vi "Process.vi"(8 "error in":errorcluster, 11 "Inst UI.SPC":refnum<class "Inst UI.SPC.lvclass">) -> (0 "error out":errorcluster, 3 "Inst UI.SPC out":refnum<class "Inst UI.SPC.lvclass">)   [LabVIEW 2019, in "Inst UI.SPC.lvclass"]
doc: "---------------------------------------------------------------\nJKI State Machine Objects™\nhttp://jki.net/state-machine-objects/\nCopyright (C) 2005-2015, JKI <info@jki.net>\nALL RIGHTS RESERVEDJKI State Machine Objects (SMO) 1.0.0.5\nJKI - JKI\nCopyright (c) 2016, JKI"
uses:
  Inst UI.SPC.lvclass
  <vilib>/JKI/JKI SMO/SMO/SMO.lvclass
  <vilib>/JKI/JKI SMO/SMO.UI/SMO.UI.lvclass
  <userlib>/LevyLab/Instrument Framework/SMOs/Instrument/Instrument.lvclass
  Inst.SPC/Typedefs/Inst.SPC.getAll--Cluster.ctl
  Inst.SPC/Inst.SPC.lvclass
  <userlib>/LevyLab/Instrument Framework/SMOs/Instrument UI/Instrument UI.lvclass
  Inst UI.SPC.UI--Cluster.ctl
  <userlib>/LevyLab/Instrument Framework/SMOs/Configuration/Configuration.lvclass
  Inst.SPC/Typedefs/Inst.SPC.Configuration--Cluster.ctl
  <userlib>/LevyLab/Instrument Framework/SMOs/Instrument/Typedefs/Client Type--Enum.ctl
  <userlib>/LevyLab/Instrument Framework/SMOs/RemoteControl/Typedefs/Message--Cluster.ctl
  <userlib>/LevyLab/Instrument Framework/SMOs/RemoteControl/RemoteControl.lvclass
  09e9697b-516c-49fb-b2dc-692589121b6f.vi
  C:/Program Files (x86)/National Instruments/LabVIEW 2019/user.lib/LevyLab/Instrument Framework/SMOs/Instrument UI/Instrument UI.lvclass
  C:/Program Files (x86)/National Instruments/LabVIEW 2019/vi.lib/JKI/JKI SMO/SMO.UI/SMO.UI.lvclass
  C:/Program Files (x86)/National Instruments/LabVIEW 2019/vi.lib/JKI/JKI SMO/SMO/SMO.lvclass
  C:/Program Files (x86)/National Instruments/LabVIEW 2019/user.lib/LevyLab/Instrument Framework/Instrument Types/VSource/Instrument.VSource.lvclass
  C:/Program Files (x86)/National Instruments/LabVIEW 2019/user.lib/LevyLab/Instrument Framework/SMOs/Instrument/Instrument.lvclass
panel:
  out "DummyData":string
  out "SPC":string
  out "DCC":string
  in  "GetConfig":bool
  in  "Parameter 2":string
  out "Counter":u32
  in  "Set Parameter":bool
  in  "Parameter":dbl
  in  "STOP":bool
  # "Connected Modules"
  # "DCC"
  # "SPC"
  # "SMO UI Template"
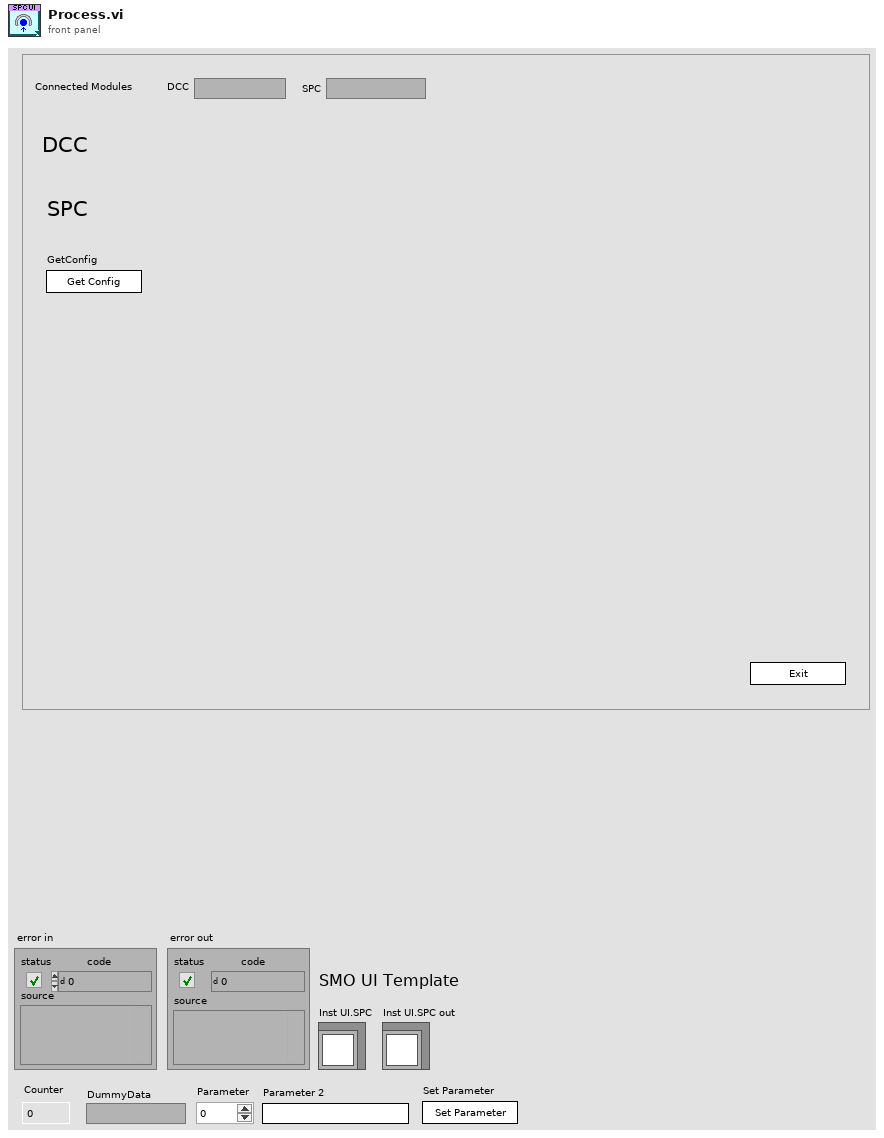
[diagram p1: front panel]
types:
  T1 = typedef "Inst.SPC.lvclass/Inst.SPC.Configuration--Cluster.ctl" = cluster{"DCC_DLL":path, "SPC_DLL":path, "DCC_Serials":string[], "SPC_Serials":string[]}
  T2 = enum32{"invalid app kind", "Development System", "Run Time System", "Student Edition", "Embedded LabVIEW", "Evaluation", "Custom"}
  T3 = enum32{"Invalid", "Standard", "Closed", "Hidden", "Minimized", "Maximized"}
  T4 = typedef "Instrument.lvclass/Client Type--Enum.ctl" = enum16{"Remote", "Local"}
  T5 = typedef "Inst.SPC.lvclass/Inst.SPC.getAll--Cluster.ctl" = cluster{"DummyData":string}
  T6 = typedef "Inst UI.SPC.lvclass/Inst UI.SPC.UI--Cluster.ctl" = cluster{"Parameter":dbl, "Parameter 2":string}
  T7 = typedef "RemoteControl.lvclass/Message--Cluster.ctl" = cluster{"Command":string, "Data":variant, "ID":string}
  T8 = cluster{"Core":cluster{"Current VI Reference":refnum<vi>, "Close Panel on Exit?":bool, "Last Error":cluster{"error":errorcluster, "previous state":string, "remaining states":string}, "Shutdown?":bool}, "Instrument UI":refnum<class "Inst UI.SPC.lvclass">, "Instrument":refnum<class "Inst.SPC.lvclass">, "Configuration":refnum<class "Configuration.lvclass">, "Config Cluster":T1, "getAll":T5, "UI Cluster":T6, "Message":T7}
  T9 = cluster{"Current VI Reference":refnum<vi>, "Close Panel on Exit?":bool, "Last Error":cluster{"error":errorcluster, "previous state":string, "remaining states":string}, "Shutdown?":bool}
  T10 = typedef "SMO.lvclass/Protected Events.ctl" = cluster{"StopProcesses":refnum<user-event>, "AbortProcesses":refnum<user-event>, "Config Changed":refnum<user-event>, "Dependency":refnum<user-event>}
  T11 = typedef "Instrument.lvclass/PublicEvents--Cluster.ctl" = cluster{"MessageFromProcess":refnum<user-event>}
  T12 = typedef "Inst.SPC.lvclass/PublicEvents--Cluster.ctl" = cluster{"MessageFromProcess":refnum<user-event>}
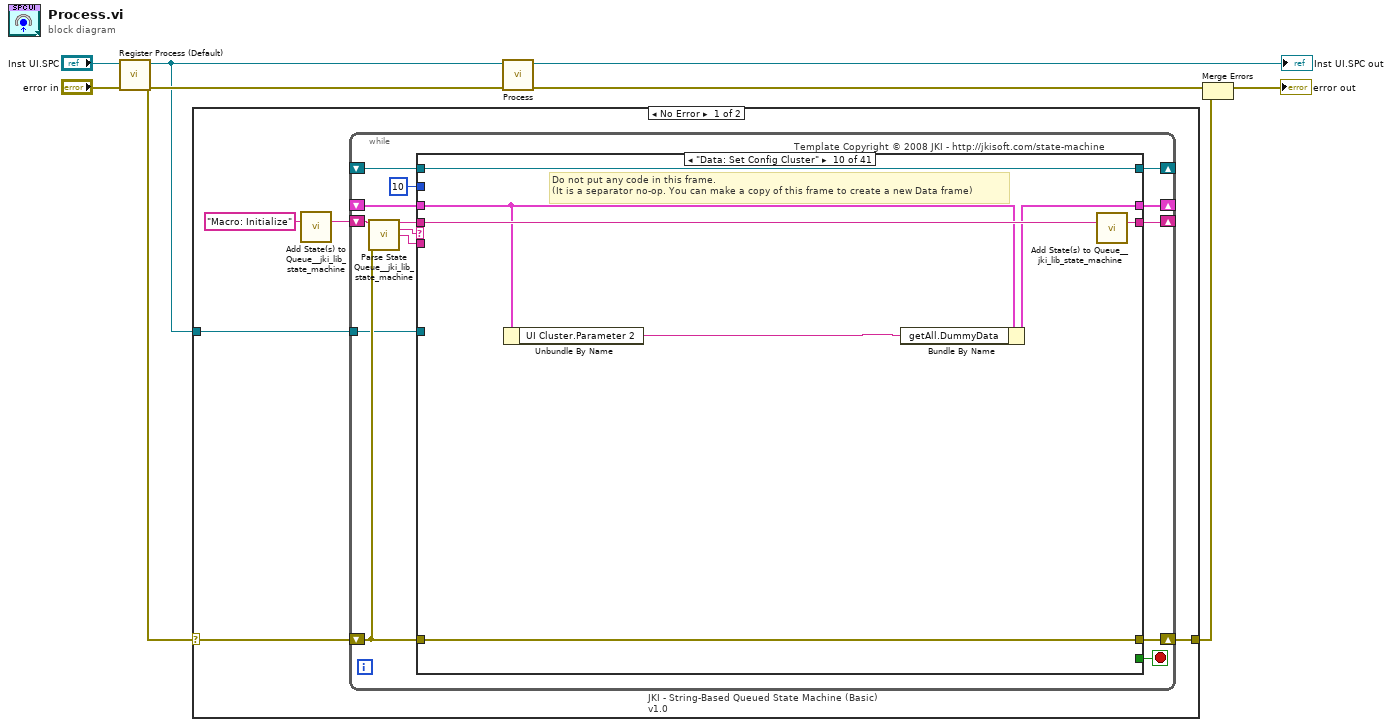
[diagram p0: block diagram]
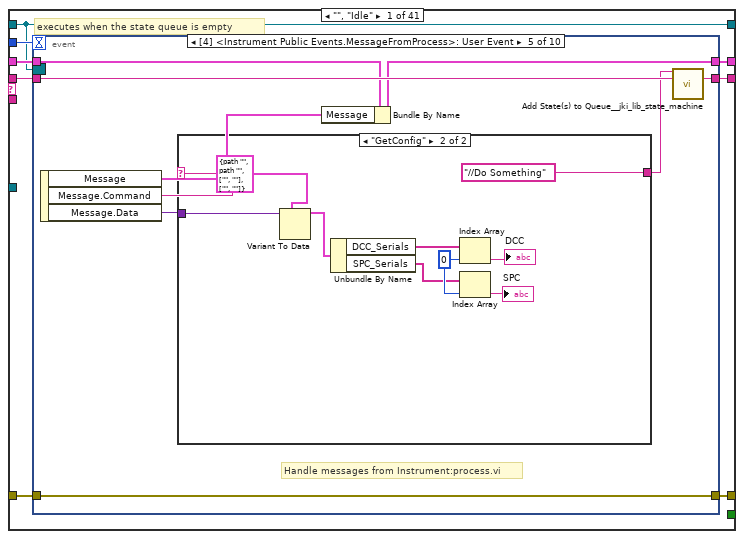
[diagram p2: hidden frame]
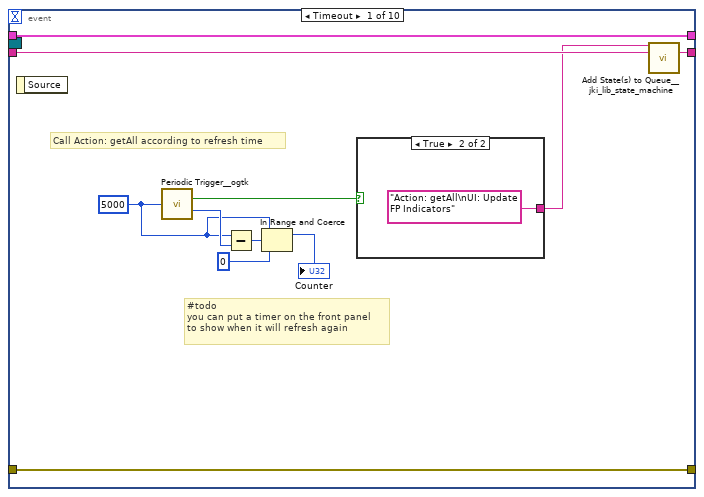
[diagram p3: hidden frame]
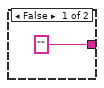
[diagram p4: hidden frame]
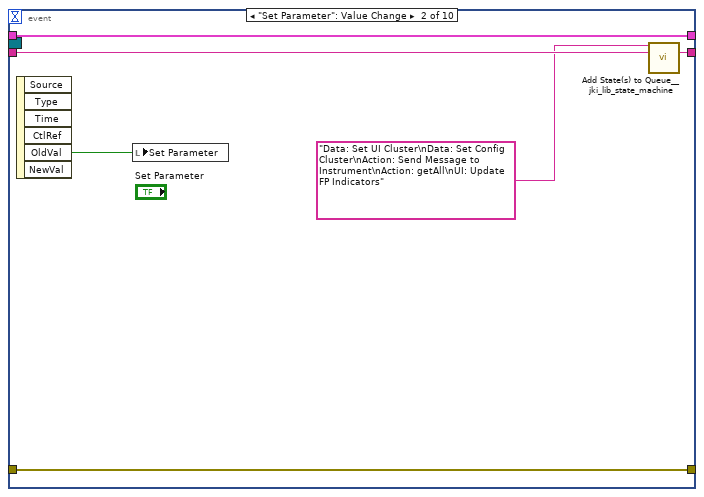
[diagram p5: hidden frame]
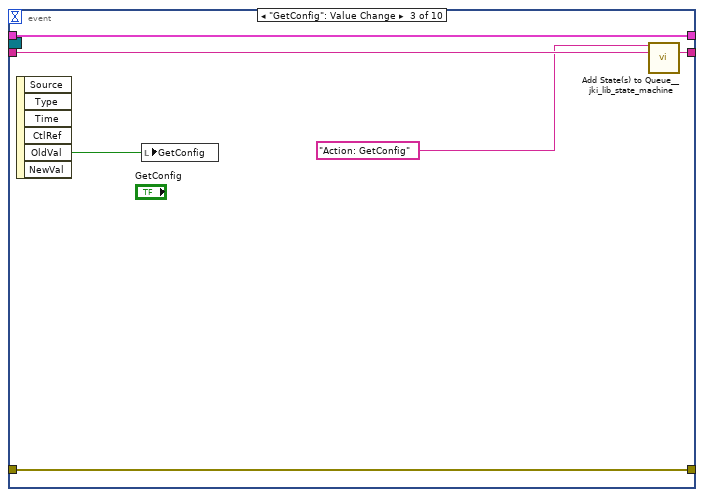
[diagram p6: hidden frame]
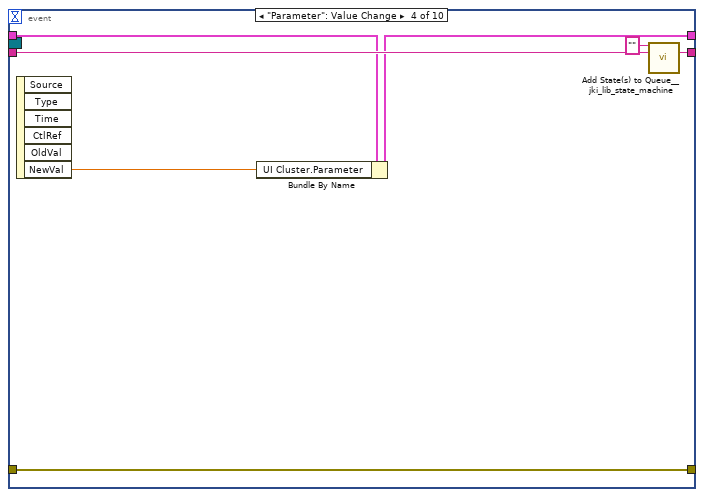
[diagram p7: hidden frame]
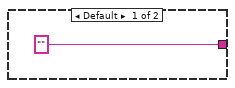
[diagram p8: hidden frame]
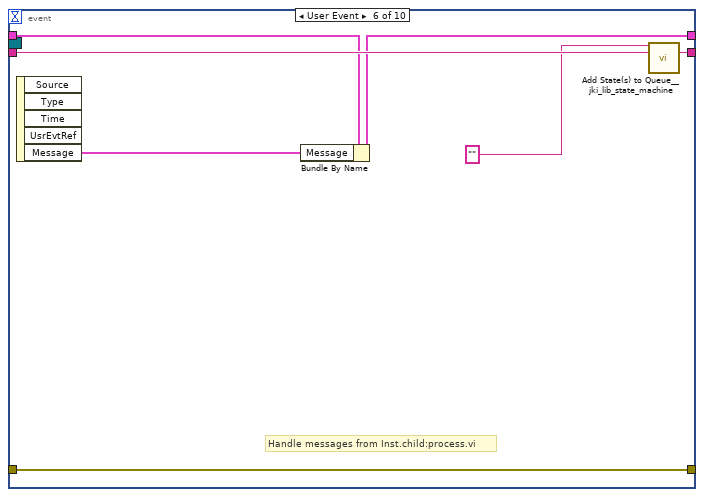
[diagram p9: hidden frame]
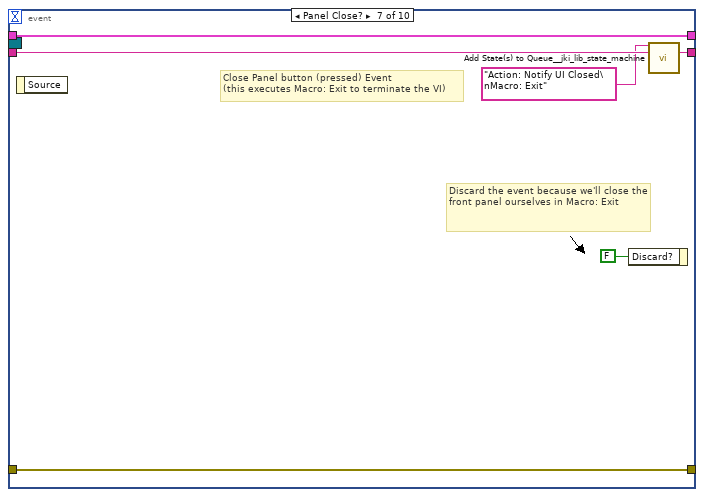
[diagram p10: hidden frame]
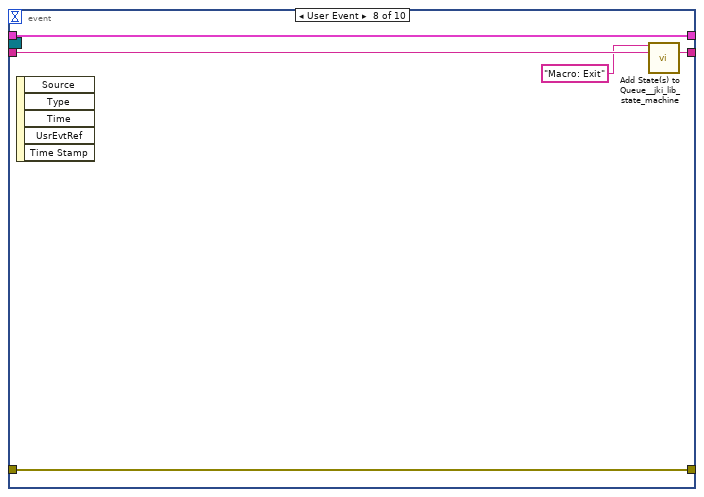
[diagram p11: hidden frame]
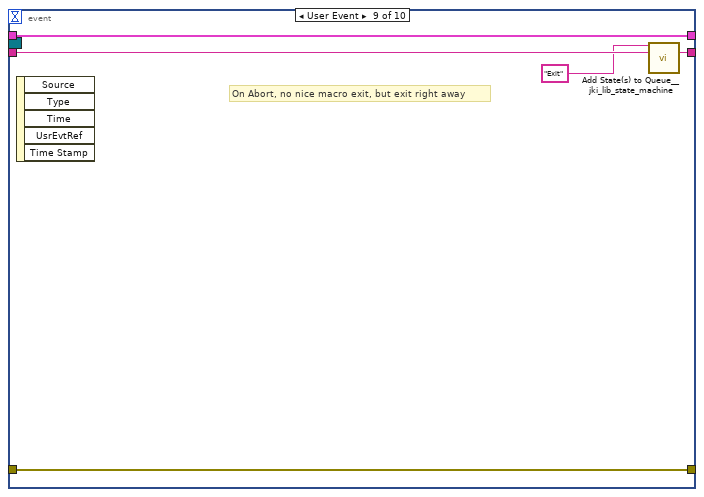
[diagram p12: hidden frame]
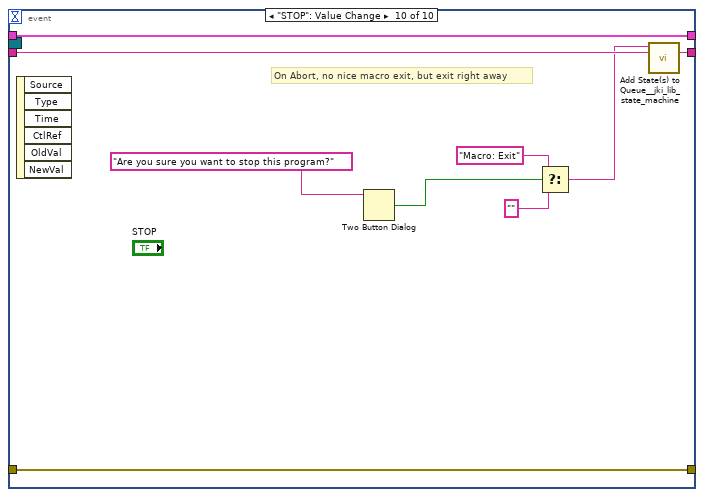
[diagram p13: hidden frame]
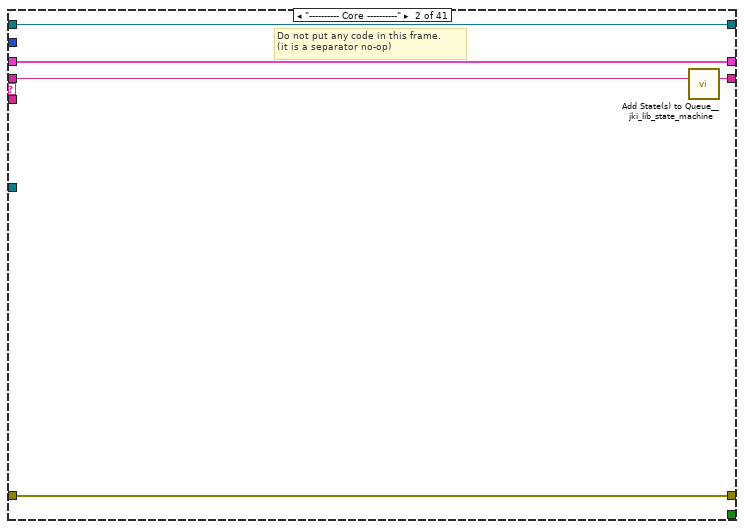
[diagram p14: hidden frame]
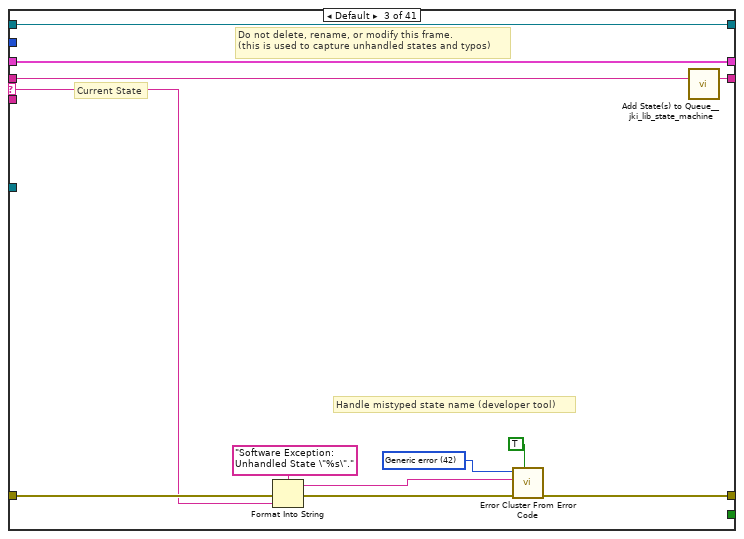
[diagram p15: hidden frame]
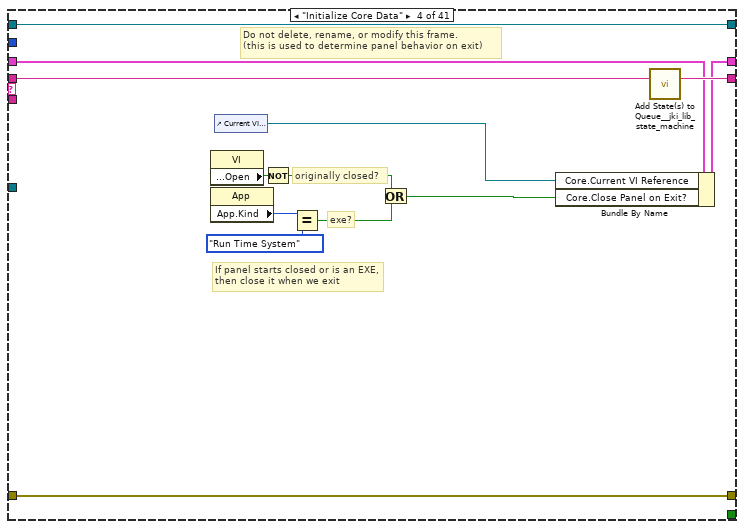
[diagram p16: hidden frame]
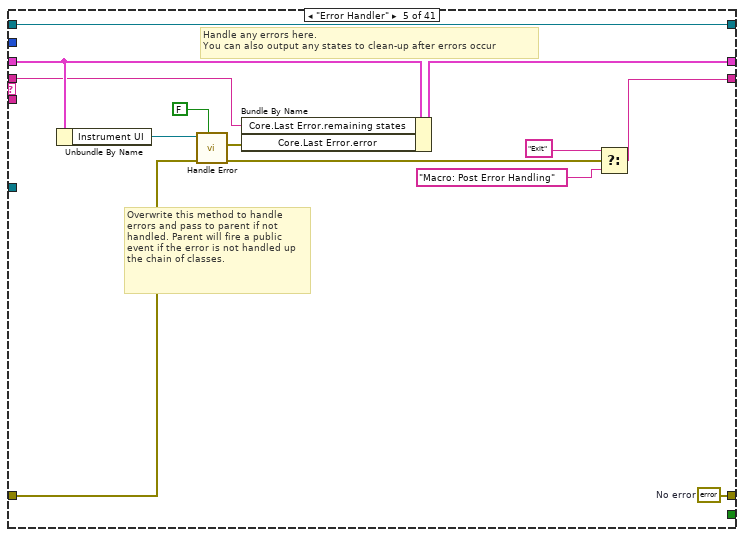
[diagram p17: hidden frame]
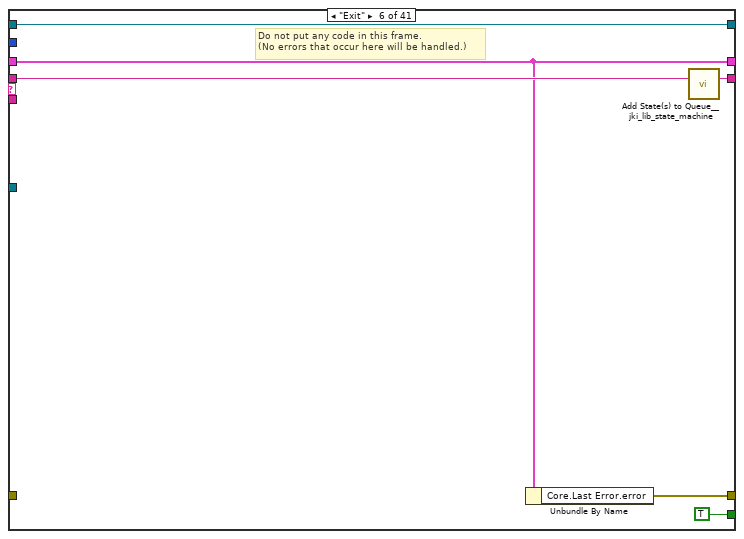
[diagram p18: hidden frame]
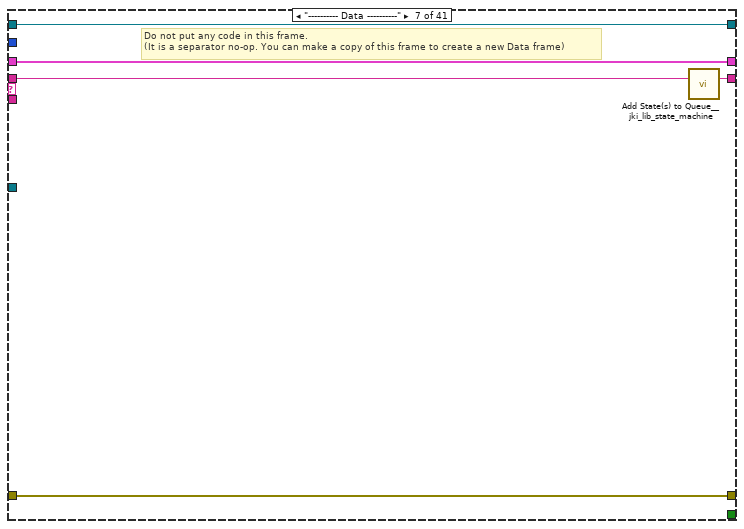
[diagram p19: hidden frame]
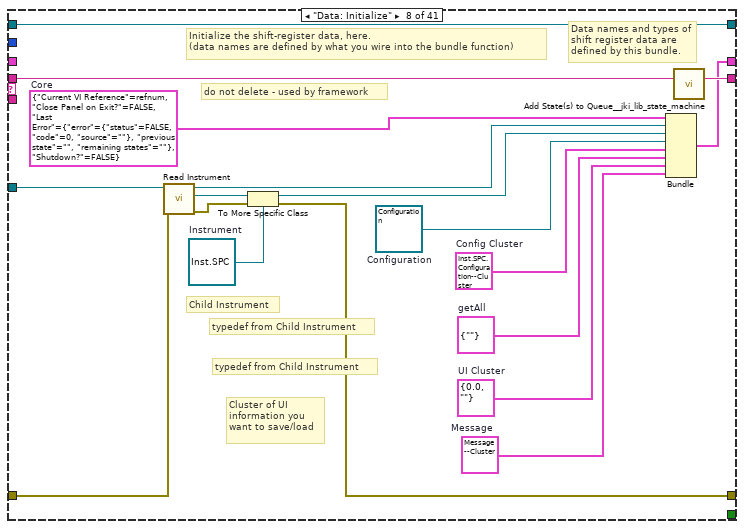
[diagram p20: hidden frame]
diagram:
  n1 = call <vilib>:"Register Process (Default).vi"("error in (no error)"="error in", "SMO"="Inst UI.SPC") -> ("error out"=w5:errorcluster, "SelfRef"=w4:refnum<class "Inst UI.SPC.lvclass">)  [unwired: 8 in]
  n2 = case shown="No Error" w5 {
    selector: w5 -> [w10 w516]
    tunnel: w4 -> [w11 _]
    tunnel: [w9 w516] -> w1
    frame No Error {
      n3 = call <vilib>:"Add State(s) to Queue__jki_lib_state_machine.vi"("State(s) in (\"\")"="Macro: Initialize") -> ("States Out"=w13:string)  [unwired: 14 in]
      n4 = while "JKI - String-Based Queued State Machine (Basic) v1.0" {
        shift-right: [w20] -> _
        shift-left: _ -> [w19]
        shift-right: [w23] -> w9
        shift-left: w10 -> [w17]
        shift-right: [w22] -> _
        shift-left: w13 -> [w24]
        tunnel: w11 -> [w16]
        shift-right: [w15] -> _
        shift-left: _ -> [w14]
        stop <- w21 stop-if-true
        # "Template Copyright © 2008 JKI - http://jkisoft.com/state-machine"
        n5 = call <vilib>:"Parse State Queue__jki_lib_state_machine.vi"("State Queue"=w24, "Error In (no error)"=w17) -> ("Remaining States"=w26:string, "Current State"=w27:string, "Arguments"=w25:string)  [unwired: 11 in]
        n6 = case shown="\"Data: Set Config Cluster\"" w27 {
          selector: w27 -> [_ _ w125 _ _ _ _ _ _ _ _ _ _ _ _ _ _ _ _ _ _ _ _ _ _ _ _ _ _ _ _ _ _ _ _ _ _ _ _ _ _]
          tunnel: w26 -> [w35 w123 w129 w148 w152 w167 w172 w190 w198 w205 w212 w217 w224 w231 w238 w245 w261 w293 w302 w314 w324 w330 w345 w350 w361 w368 w373 w389 w395 w400 w415 w423 w435 w442 w449 w461 w474 w484 w494 w504 w515]
          tunnel: w25 -> [_ _ _ _ _ _ _ _ _ _ _ _ _ _ _ w239 w255 _ _ _ _ _ _ _ _ _ _ _ _ _ _ _ _ _ _ _ _ _ _ _ _]
          tunnel: w19 -> [w33 w120 w127 w139 w155 w163 w169 _ w194 w201 w206 w214 w222 w227 w233 w243 w257 w290 w298 w304 w321 w327 w332 w347 w358 w363 w370 w387 w393 w397 w408 w420 w426 w437 w443 w453 w468 w476 w489 w499 w511]
          tunnel: [w32 w121 w131 w145 w157 w162 w170 w177 w196 w203 w208 w215 w219 w229 w234 w240 w258 w291 w300 w312 w322 w328 w343 w348 w352 w364 w371 w384 w390 w398 w401 w418 w427 w439 w444 w458 w471 w481 w485 w495 w505] -> w23
          tunnel: w17 -> [w31 w121 w130 w145 w151 _ w170 w174 w196 w203 w209 w215 w220 w229 w234 w241 w259 w291 w300 w312 w322 w328 w343 w348 w353 w365 w371 w374 w391 w398 w410 w416 w428 w439 w445 w454 w463 w477 w486 w496 w506]
          tunnel: [w34 w122 w128 w147 w149 w166 w171 w189 w197 w204 w211 w216 w223 w230 w237 w244 w260 w292 w301 w313 w323 w329 w344 w349 w360 w367 w372 w388 w394 w399 w414 w422 w434 w441 w448 w460 w473 w483 w493 w503 w514] -> w22
          tunnel: [_ _ _ _ _ TRUE _ _ _ _ _ _ _ _ _ _ _ _ _ _ _ _ _ _ _ _ _ _ _ _ _ _ _ _ _ _ _ _ _ _ _] -> w21
          tunnel: [w30 w120 w127 w146 w154 w163 w169 w188 w193 w200 w206 w214 w222 w227 w233 w243 w257 w290 w298 w305 w321 w327 w332 w347 w358 w363 w370 w387 w393 w397 w412 w420 w424 w436 w443 w455 w469 w478 w490 w500 w510] -> w20
          tunnel: 10 ("Timeout") -> [w29 _ _ _ _ _ _ _ _ _ _ _ _ _ _ _ _ _ _ _ _ _ _ _ _ _ _ _ _ _ _ _ _ _ _ _ _ _ _ _ _]
          tunnel: w16 -> [_ _ _ _ _ _ _ w175 _ _ _ _ _ _ _ _ _ _ _ _ _ _ _ _ _ _ _ _ _ _ _ _ _ _ _ _ _ _ _ _ _]
          tunnel: [w28 w119 w124 w136 w161 w164 w168 w187 w195 w202 w207 w213 w221 w228 w236 w242 w254 w289 w299 w311 w320 w326 w337 w346 w359 w366 w369 w386 w392 w396 w413 w421 w433 w440 w447 w459 w472 w482 w492 w502 w513] -> w15
          tunnel: w14 -> [w28 w119 w124 w136 w161 w164 w168 w187 w195 w202 w207 w213 w221 w228 w236 w242 w254 w289 w299 w311 w320 w326 w337 w346 w359 w366 w369 _ w392 w396 w413 w421 w433 w440 w447 w459 w472 w482 w492 w502 w513]
          frame "", "Idle" {
            # "executes when the state queue is empty"
            n7 = event shown="[4] <Instrument Public Events.MessageFromProcess>: User Event" {
              selector: w28 -> [_ _ _ _ _ _ _ _ _ _]
              dyn-events: _ -> [_ _ _ _ _ _ _ _ _ _]
              timeout: w29 -> [_ _ _ _ _ _ _ _ _ _]
              tunnel: w35 -> [w46 w54 w60 w67 w76 w93 w99 w104 w109 w118]
              tunnel: [w45 w53 w59 w66 w75 w92 w98 w103 w108 w117] -> w34
              tunnel: w33 -> [w43 w51 w57 w63 w73 w90 w95 w101 w106 w115]
              tunnel: [w44 w52 w58 w65 w74 w91 w94 w102 w107 w116] -> w32
              tunnel: w31 -> [w44 w52 w58 w65 w74 w91 w94 w102 w107 w116]
              tunnel: [w43 w51 w57 w62 w72 w89 w95 w101 w106 w115] -> w30
              event Timeout {
                w37 = u32 5000 ("time (ms)")
                # "#todo\nyou can put a timer on the front panel\nto show when it will refresh again"
                # "Call Action: getAll according to refresh time"
                n8 = event-data() -> ()  [unwired: 1 in, 1 out]
                n9 = call <userlib>:"Periodic Trigger__ogtk.vi"("time (ms)"=w37) -> ("Triggered"=w41:bool, "timer value"=w40:u32)  [unwired: 12 in, 1 out]
                n10 = Subtract(x=w37, y=w40) -> (x-y=w39:u32)
                n11 = In Range and Coerce(upper limit=w37, x=w39, lower limit=u32 0) -> (coerced(x)=→"Counter":u32)  [unwired: 1 out]
                n12 = case shown="True" w41 {
                  tunnel: ["" ("State(s) in Front (\"\")") "Action: getAll\nUI: Update FP Indicators" ("State(s) in Front (\"\")")] -> w42
                  frame False {
                  }
                  frame True {
                  }
                }
                n13 = call <vilib>:"Add State(s) to Queue__jki_lib_state_machine.vi"("State(s) in Front (\"\")"=w42, "State(s) in (\"\")"=w46) -> ("States Out"=w45:string)  [unwired: 13 in]
              }
              event "Set Parameter": Value Change {
                n14 = event-data() -> ("OldVal"=w50:bool)  [unwired: 1 in, 5 out]
                n15 = local write "Set Parameter"(w50) -> ()
                n16 = call <vilib>:"Add State(s) to Queue__jki_lib_state_machine.vi"("State(s) in Front (\"\")"="Data: Set UI Cluster\nData: Set Config Cluster\nAction: Send Message to Instrument\nAction: getAll\nUI: Update FP Indicators" ("State(s) in Front (\"\")"), "State(s) in (\"\")"=w54) -> ("States Out"=w53:string)  [unwired: 13 in]
              }
              event "GetConfig": Value Change {
                n17 = event-data() -> ("OldVal"=w56:bool)  [unwired: 1 in, 5 out]
                n18 = local write "GetConfig"(w56) -> ()
                n19 = call <vilib>:"Add State(s) to Queue__jki_lib_state_machine.vi"("State(s) in Front (\"\")"="Action: GetConfig" ("State(s) in Front (\"\")"), "State(s) in (\"\")"=w60) -> ("States Out"=w59:string)  [unwired: 13 in]
              }
              event "Parameter": Value Change {
                n20 = event-data() -> ("NewVal"=w64:dbl)  [unwired: 1 in, 5 out]
                n21 = Bundle By Name(cluster=w63, "UI Cluster.Parameter"=w64) -> (w62:T8)
                n22 = call <vilib>:"Add State(s) to Queue__jki_lib_state_machine.vi"("State(s) in Front (\"\")"="" ("State(s) in Front (\"\")"), "State(s) in (\"\")"=w67) -> ("States Out"=w66:string)  [unwired: 13 in]
              }
              event User Event {
                # "Handle messages from Instrument:process.vi"
                n23 = event-data() -> ("Message"=w70:T7, "Message.Command"=w69:string, "Message.Data"=w68:variant)  [unwired: 1 in]
                n24 = case shown="\"GetConfig\"" w69 {
                  tunnel: ["" ("State(s) in Front (\"\")") "//Do Something" ("State(s) in Front (\"\")")] -> w71
                  tunnel: w68 -> [_ w85]
                  frame Default {
                  }
                  frame "GetConfig" {
                    w81 = 0 ("index")
                    n25 = Variant To Data(type=T1 {"DCC_DLL"=path "", "SPC_DLL"=path "", "DCC_Serials"=["", ""], "SPC_Serials"=["", ""]} ("Configuration"), Variant=w85) -> (data=w84:T1)  [unwired: 1 in, 1 out]
                    n26 = Unbundle By Name(w84) -> ("DCC_Serials"=w83:string[], "SPC_Serials"=w80:string[])
                    n27 = Index Array(array=w83, index=w81) -> (element=→"DCC":string)
                    n28 = Index Array(array=w80, index=w81) -> (element=→"SPC":string)
                  }
                }
                n29 = Bundle By Name(cluster=w73, "Message"=w70) -> (w72:T8)
                n30 = call <vilib>:"Add State(s) to Queue__jki_lib_state_machine.vi"("State(s) in Front (\"\")"=w71, "State(s) in (\"\")"=w76) -> ("States Out"=w75:string)  [unwired: 13 in]
              }
              event User Event {
                # "Handle messages from Inst.child:process.vi"
                n31 = event-data() -> ("Message"=w87:T7)  [unwired: 1 in, 4 out]
                n32 = Bundle By Name(cluster=w90, "Message"=w87) -> (w89:T8)
                n33 = call <vilib>:"Add State(s) to Queue__jki_lib_state_machine.vi"("State(s) in Front (\"\")"="" ("State(s) in Front (\"\")"), "State(s) in (\"\")"=w93) -> ("States Out"=w92:string)  [unwired: 13 in]
              }
              event Panel Close? {
                # "Discard the event because we'll close the front panel ourselves in Macro: Exit"
                # "Close Panel button (pressed) Event\n(this executes Macro: Exit to terminate the VI)"
                n34 = event-data() -> ()  [unwired: 1 in, 1 out]
                n35 = event-data("Discard?"=FALSE) -> ()  [unwired: 1 in, 1 out]
                n36 = call <vilib>:"Add State(s) to Queue__jki_lib_state_machine.vi"("State(s) in Front (\"\")"="Action: Notify UI Closed\nMacro: Exit", "State(s) in (\"\")"=w99) -> ("States Out"=w98:string)  [unwired: 13 in]
              }
              event User Event {
                n37 = event-data() -> ()  [unwired: 1 in, 5 out]
                n38 = call <vilib>:"Add State(s) to Queue__jki_lib_state_machine.vi"("State(s) in Front (\"\")"="Macro: Exit", "State(s) in (\"\")"=w104) -> ("States Out"=w103:string)  [unwired: 13 in]
              }
              event User Event {
                # "On Abort, no nice macro exit, but exit right away"
                n39 = event-data() -> ()  [unwired: 1 in, 5 out]
                n40 = call <vilib>:"Add State(s) to Queue__jki_lib_state_machine.vi"("State(s) in Front (\"\")"="Exit", "State(s) in (\"\")"=w109) -> ("States Out"=w108:string)  [unwired: 13 in]
              }
              event "STOP": Value Change {
                # "On Abort, no nice macro exit, but exit right away"
                n41 = event-data() -> ()  [unwired: 1 in, 6 out]
                n42 = Two Button Dialog(message="Are you sure you want to stop this program?") -> (T button?=w114:bool)  [unwired: 2 in]
                n43 = Select(t="Macro: Exit", s=w114, f="") -> (s? t:f=w110:string)
                n44 = call <vilib>:"Add State(s) to Queue__jki_lib_state_machine.vi"("State(s) in Front (\"\")"=w110, "State(s) in (\"\")"=w118) -> ("States Out"=w117:string)  [unwired: 13 in]
              }
            }
          }
          frame "---------- Core ----------" {
            # "Do not put any code in this frame.\n(it is a separator no-op)"
            n45 = call <vilib>:"Add State(s) to Queue__jki_lib_state_machine.vi"("State(s) in (\"\")"=w123) -> ("States Out"=w122:string)  [unwired: 14 in]
          }
          frame Default {
            w134 = 42 items=["No error", "Argument error", "Memory is full", "Out of zone", "End of file", "File already open", "Generic file I/O error", "File not found", "File permission error", "Disk is full", "Duplicate path", "Too many files open", "System feature not enabled", "Resource file not found", "Cannot add resource", "Resource not found", "Image not found", "Image memory error", "Pen does not exist", "Config type invalid", "Config token not found", "Config parse error", "Config memory error", "Bad external code format", "Bad external code offset", "External code not present", "Null window", "Destroy window error", "Null menu", "Print aborted", "Bad print record", "Print driver error", "Windows error during printing", "Memory error during printing", "Print dialog error", "Generic print error", "Invalid device refnum", "Device not found", "Device parameter error", "Device unit error", "Cannot open device", "Device call aborted", "Generic error", "Cancelled by user", "Object ID too low", "Object ID too high", "Object not in heap", "Unknown heap", "Unknown object (invalid DefProc)", "Unknown object (DefProc not in table)", "Message out of range", "Invalid (null) method", "Unknown message", "Manager call not supported", "Bad address", "Network operation in progress", "Network operation timed out", "Connection is busy", "Network attribute not supported", "Network error", "Address in use", "System out of memory", "Connection aborted", "Connection refused", "Not connected", "Already connected", "Connection closed", "Initialization error (interapplication manager)", "Bad occurrence", "Wait on unbound occurrence handler", "Occurrence queue overflow", "Datalog type conflict", "Unused", "Unrecognized type (interapplication manager)", "Memory corrupt", "Failed to make temporary DLL", "Old CIN version", "Drag socket not found", "Failed to load drop-object", "Failed to register OLE object", "Failed to release OLE object", "Format specifier type mismatch", "Unknown format specifier", "Too few format specifiers", "Too many format specifiers", "Scan failed", "Newer CIN version", "Error converting to variant", "Runtime menu error", "Password tampered", "Variant attribute not found", "Incompatible variant data type", "Event data is not available", "Event Store is not present", "Occurrence is not found", "Event Queue is not created", "Event info is not available", "Refnum passed is NULL", "Error retrieving Class GUID", "Error retrieving CoClass GUID", "Error retrieving TypeLib GUID.", "Bad built application magic bytes.", "Specific driver is different from the specific driver associated with the Logical Name.", "There is no session opened to the class driver.", "Max Error", "MAX - Error with config objects", "MAX - Error loading configuration", "MAX - Group not supported"]
            # "Current State"
            # "Do not delete, rename, or modify this frame.\n(this is used to capture unhandled states and typos)"
            # "Handle mistyped state name (developer tool)"
            n46 = Format Into String(format string="Software Exception: Unhandled State \"%s\"." ("message"), error in=w130, w125) -> (resulting string=w133:string, error out=w132:errorcluster)  [unwired: 1 in]
            n47 = call <vilib>:"Error Cluster From Error Code.vi"("show call chain? (False)"=TRUE, "error in (no error)"=w132, "error message (\"\")"=w133, "error code (0)"=w134) -> ("error out"=w131:errorcluster)  [unwired: 5 in]
            n48 = call <vilib>:"Add State(s) to Queue__jki_lib_state_machine.vi"("State(s) in (\"\")"=w129) -> ("States Out"=w128:string)  [unwired: 14 in]
          }
          frame "Initialize Core Data" {
            # "Do not delete, rename, or modify this frame.\n(this is used to determine panel behavior on exit)"
            # "originally closed?"
            # "exe?"
            # "If panel starts closed or is an EXE, then close it when we exit"
            n49 = property class="VI"() -> ("Front Panel.Open"=w144:bool)  [unwired: 2 in, 2 out]
            n50 = property class="App"() -> ("App.Kind"=w143:T2)  [unwired: 2 in, 2 out]
            n51 = control-ref of="Current VI Reference"() -> (w137:refnum<vi>)
            n52 = Not(x=w144) -> (.not. x?=w141:bool)
            n53 = Equal?(x=w143, y=T2."Run Time System" ("Application:Kind")) -> (x = y?=w140:bool)
            n54 = Or(x=w141, y=w140) -> (x .or. y?=w138:bool)
            n55 = Bundle By Name(cluster=w139, "Core.Current VI Reference"=w137, "Core.Close Panel on Exit?"=w138) -> (w146:T8)
            n56 = call <vilib>:"Add State(s) to Queue__jki_lib_state_machine.vi"("State(s) in (\"\")"=w148) -> ("States Out"=w147:string)  [unwired: 14 in]
          }
          frame "Error Handler" {
            w157 = errorcluster {"status"=FALSE, "code"=0, "source"=""}  # No error
            # "Overwrite this method to handle errors and pass to parent if not handled. Parent will fire a public event if the error is not handled up the chain of classes."
            # "Handle any errors here.\nYou can also output any states to clean-up after errors occur"
            n57 = Unbundle By Name(w155) -> ("Instrument UI"=w160:refnum<class "Inst UI.SPC.lvclass">)
            n58 = call-dynamic "Handle Error.vi"("Stop on Unhandled Error (T)"=FALSE, "error in"=w151, "SMO"=w160) -> ("handling error"=w158:errorcluster, "Unhandled error"=w156:errorcluster)  [unwired: 6 in, 1 out]
            n59 = Bundle By Name(cluster=w155, "Core.Last Error.remaining states"=w152, "Core.Last Error.error"=w156) -> (w154:T8)
            n60 = Select(t="Exit", s=w158, f="Macro: Post Error Handling") -> (s? t:f=w149:string)
          }
          frame "Exit" {
            # "Do not put any code in this frame.\n(No errors that occur here will be handled.)"
            n61 = Unbundle By Name(w163) -> ("Core.Last Error.error"=w162:errorcluster)
            n62 = call <vilib>:"Add State(s) to Queue__jki_lib_state_machine.vi"("State(s) in (\"\")"=w167) -> ("States Out"=w166:string)  [unwired: 14 in]
          }
          frame "---------- Data ----------" {
            # "Do not put any code in this frame.\n(It is a separator no-op. You can make a copy of this frame to create a new Data frame)"
            n63 = call <vilib>:"Add State(s) to Queue__jki_lib_state_machine.vi"("State(s) in (\"\")"=w172) -> ("States Out"=w171:string)  [unwired: 14 in]
          }
          frame "Data: Initialize" {
            w173 = T7 {"Command"="", "Data"=variant, "ID"=""}  # Message
            w176 = refnum<class "Configuration.lvclass"> refnum  # Configuration
            w179 = T1 {"DCC_DLL"=path "C:/Program Files (x86)/BH/SPCM/DLL/spcm64.dll", "SPC_DLL"=path "C:/Program Files (x86)/BH/SPCM/DLL/spcm64.dll", "DCC_Serials"=["", ""], "SPC_Serials"=["", ""]}  # Config Cluster
            w181 = T6 {"Parameter"=0.0, "Parameter 2"=""}  # UI Cluster
            w183 = refnum<class "Inst.SPC.lvclass"> refnum  # Instrument
            w185 = T5 {"DummyData"=""}  # getAll
            w186 = T9 {"Current VI Reference"=refnum, "Close Panel on Exit?"=FALSE, "Last Error"={"error"={"status"=FALSE, "code"=0, "source"=""}, "previous state"="", "remaining states"=""}, "Shutdown?"=FALSE}  # Core
            # "typedef from Child Instrument"
            # "Cluster of UI\ninformation you\nwant to save/load"
            # "Child Instrument"
            # "typedef from Child Instrument"
            # "do not delete - used by framework"
            # "Data names and types of shift register data are defined by this bundle."
            # "Initialize the shift-register data, here.\n(data names are defined by what you wire into the bundle function)"
            n64 = call <userlib>:"Read Instrument.vi"("error in (no error)"=w174, "Instrument UI in"=w175) -> ("error out"=w180:errorcluster, "Instrument"=w182:refnum<class "Instrument.lvclass">, "Instrument UI"=w184:refnum<class "Inst UI.SPC.lvclass">)  [unwired: 7 in]
            n65 = To More Specific Class(target class=w183, reference=w182, error in=w180) -> (specific class reference=w178:refnum<class "Inst.SPC.lvclass">, error out=w177:errorcluster)
            n66 = Bundle("Core"=w186, "Instrument UI"=w184, "Instrument"=w178, "Configuration"=w176, "Config Cluster"=w179, "getAll"=w185, "UI Cluster"=w181, "Message"=w173) -> (w188:T8)  [unwired: 1 in]
            n67 = call <vilib>:"Add State(s) to Queue__jki_lib_state_machine.vi"("State(s) in (\"\")"=w190) -> ("States Out"=w189:string)  [unwired: 14 in]
          }
          frame "Data: Set UI Cluster" {
            # "Do not put any code in this frame.\n(It is a separator no-op. You can make a copy of this frame to create a new Data frame)"
            n68 = Bundle By Name(cluster=w194, "UI Cluster.Parameter"="Parameter", "UI Cluster.Parameter 2"="Parameter 2") -> (w193:T8)
            n69 = call <vilib>:"Add State(s) to Queue__jki_lib_state_machine.vi"("State(s) in (\"\")"=w198) -> ("States Out"=w197:string)  [unwired: 14 in]
          }
          frame "Data: Set Config Cluster" {
            # "Do not put any code in this frame.\n(It is a separator no-op. You can make a copy of this frame to create a new Data frame)"
            n70 = Unbundle By Name(w201) -> ("UI Cluster.Parameter 2"=w199:string)
            n71 = Bundle By Name(cluster=w201, "getAll.DummyData"=w199) -> (w200:T8)
            n72 = call <vilib>:"Add State(s) to Queue__jki_lib_state_machine.vi"("State(s) in (\"\")"=w205) -> ("States Out"=w204:string)  [unwired: 14 in]
          }
          frame "Data: Cleanup" {
            # "Cleanup any data and references, here.\n(this is called automatically, by the Macro: Exit)"
            n73 = Unbundle By Name(w206) -> ("Core.Current VI Reference"=w210:refnum<vi>)
            n74 = Close Reference(reference=w210, error in (no error)=w209) -> (error out=w208:errorcluster)
            n75 = call <vilib>:"Add State(s) to Queue__jki_lib_state_machine.vi"("State(s) in (\"\")"=w212) -> ("States Out"=w211:string)  [unwired: 14 in]
          }
          frame "---------- UI ----------" {
            # "Do not put any code in this frame.\n(It is a separator no-op. You can make a copy of this frame to create a new UI frame)"
            n76 = call <vilib>:"Add State(s) to Queue__jki_lib_state_machine.vi"("State(s) in (\"\")"=w217) -> ("States Out"=w216:string)  [unwired: 14 in]
          }
          frame "UI: Initialize" {
            # "size window to decoration box on front panel"
            # "Initialize the User Interface, here.\n(this is called automatically, by the Macro: Init)"
            n77 = invoke on="STOP" class="Bool (strict)" method="Reinit To Default"() -> ()  [unwired: 3 in, 3 out]
            n78 = call <userlib>:"Fit VI window to Largest Dec__ogtk.vi"("error in (no error)"=w220, "border spacing (2 px)"=0) -> ("error out"=w219:errorcluster)  [unwired: 4 in, 1 out]
            n79 = call <vilib>:"Add State(s) to Queue__jki_lib_state_machine.vi"("State(s) in (\"\")"=w224) -> ("States Out"=w223:string)  [unwired: 14 in]
          }
          frame "UI: Update FP Controls" {
            # "Do not put any code in this frame.\n(It is a separator no-op. You can make a copy of this frame to create a new UI frame)"
            n80 = Unbundle By Name(w227) -> ("UI Cluster.Parameter"=w225:dbl, "UI Cluster.Parameter 2"=w226:string)
            n81 = local write "Parameter 2"(w226) -> ()
            n82 = local write "Parameter"(w225) -> ()
            n83 = call <vilib>:"Add State(s) to Queue__jki_lib_state_machine.vi"("State(s) in (\"\")"=w231) -> ("States Out"=w230:string)  [unwired: 14 in]
          }
          frame "UI: Update FP Indicators" {
            # "do this way to have nicer UI or only display what you want"
            n84 = Unbundle By Name(w233) -> ("getAll"=w235:T5)
            n85 = Unbundle By Name(w235) -> ("DummyData"=→"DummyData":string)
            n86 = call <vilib>:"Add State(s) to Queue__jki_lib_state_machine.vi"("State(s) in (\"\")"=w238) -> ("States Out"=w237:string)  [unwired: 14 in]
          }
          frame "UI: Cursor Set" {
            # "Argument"
            # "Initialize the User Interface, here.\n(this is called automatically, by the Macro: Init)"
            n87 = disable-structure shown="Default" {
              disable-tunnel: w241 -> [w246 w249]
              disable-tunnel: [w246 w248] -> w240
              disable-tunnel: w239 -> [_ w247]
              frame condition #0 {
              }
              frame condition #1 (active) {
                n88 = case shown="\"Busy\"" w247 {
                  tunnel: w249 -> [w251 w253]
                  tunnel: [w250 w252] -> w248
                  frame "Idle", Default {
                    n89 = call <vilib>:"Unset Busy.vi"("error in (no error)"=w251) -> ("error out"=w250:errorcluster)  [unwired: 10 in]
                  }
                  frame "Busy" {
                    n90 = call <vilib>:"Set Busy.vi"("error in (no error)"=w253) -> ("error out"=w252:errorcluster)  [unwired: 9 in, 1 out]
                  }
                }
              }
            }
            n91 = call <vilib>:"Add State(s) to Queue__jki_lib_state_machine.vi"("State(s) in (\"\")"=w245) -> ("States Out"=w244:string)  [unwired: 14 in]
          }
          frame "UI: Front Panel State" {
            # "Argument"
            # "Set Front Panel Open or Closed\n(Usage: \"UI: Front Panel State >> Open|Close\")"
            n92 = Unbundle By Name(w257) -> ("Core.Current VI Reference"=w256:refnum<vi>)
            n93 = disable-structure shown="Default" {
              disable-tunnel: w259 -> [w265 w288]
              disable-tunnel: [w264 w288] -> w258
              disable-tunnel: w256 -> [w263 _]
              disable-tunnel: w255 -> [w262 _]
              frame condition #0 (active) {
                n94 = case shown="\"Close\"" w262 {
                  tunnel: w265 -> [w269 w282]
                  tunnel: [w271 w283] -> w264
                  tunnel: w263 -> [w270 w280]
                  frame "Open", Default {
                    n95 = property class="VI"(reference=w270, error in=w269) -> (reference out=w267:refnum<vi>, error out=w268:errorcluster, "FP.State"=w266:T3)
                    n96 = case shown="\"Closed\"" w266 {
                      tunnel: [w274 w277] -> w271
                      tunnel: w268 -> [w273 w277]
                      tunnel: w267 -> [w272 _]
                      frame "Closed" {
                        n97 = invoke class="VI" method="FP.Open"(reference=w272, error in=w273, "Activate"=TRUE, "State"=T3."Standard") -> (error out=w274:errorcluster)  [unwired: 1 in, 4 out]
                      }
                      frame Default {
                      }
                    }
                  }
                  frame "Close" {
                    n98 = property class="VI"(reference=w280, error in=w282) -> (reference out=w279:refnum<vi>, error out=w281:errorcluster, "FP.State"=w278:T3)
                    n99 = case shown="Default" w278 {
                      tunnel: [w284 w287] -> w283
                      tunnel: w281 -> [w284 w286]
                      tunnel: w279 -> [_ w285]
                      frame "Invalid", "Closed" {
                      }
                      frame Default {
                        n100 = invoke class="VI" method="FP.Close"(reference=w285, error in=w286) -> (error out=w287:errorcluster)  [unwired: 1 in, 2 out]
                      }
                    }
                  }
                }
              }
              frame condition #1 {
              }
            }
            n101 = call <vilib>:"Add State(s) to Queue__jki_lib_state_machine.vi"("State(s) in (\"\")"=w261) -> ("States Out"=w260:string)  [unwired: 14 in]
          }
          frame "---------- Macro ----------" {
            # "Do not put any code in this frame.\n(It is a separator no-op. You can make a copy of this frame to create a new Macro frame)"
            n102 = call <vilib>:"Add State(s) to Queue__jki_lib_state_machine.vi"("State(s) in (\"\")"=w293) -> ("States Out"=w292:string)  [unwired: 14 in]
          }
          frame "Macro: Initialize" {
            w296 = "UI: Initialize\nMacro: Read UI Config\nAction: Open\nAction: GetConfig\n//UI: Front Panel State >> Open"  # UI: Initialize Macro: Read UI Config Action: Open Action: GetConfig //UI: Front Panel State >> Open
            # "Initialization Macro\n(This is called once, when the VI starts)"
            n103 = call <vilib>:"Add State(s) to Queue__jki_lib_state_machine.vi"("State(s) in Front (\"\")"="Data: Initialize\nInitialize Core Data\nEvents: Register", "State(s) in (\"\")"="Process: Sync", "State(s) at Back (\"\")"=w296) -> ("States Out"=w295:string)  [unwired: 12 in]
            n104 = call <vilib>:"Add State(s) to Queue__jki_lib_state_machine.vi"("State(s) in Front (\"\")"=w295, "State(s) in (\"\")"=w302) -> ("States Out"=w301:string)  [unwired: 13 in]
          }
          frame "Macro: Post Error Handling" {
            # "Clear Last Error?"
            n105 = Unbundle By Name(w304) -> ("Core.Last Error.remaining states"=w306:string, "Core.Shutdown?"=w307:bool)
            n106 = Unbundle By Name(w304) -> ("Core.Last Error.error"=w310:errorcluster)
            n107 = case shown="False" FALSE {
              tunnel: w310 -> [w318 _]
              tunnel: [w318 _] -> w309
              frame False {
              }
              frame True {
              }
            }
            n108 = case shown="True" w307 {
              tunnel: w306 -> [w315 w317]
              tunnel: [w315 w316] -> w303
              frame False {
                # "These are the remaining states (at the moment the error occured). States can be altered according to business logic."
                # "NOT SHUTTING DOWN"
              }
              frame True {
                # "Developer can decide to alter the states but should be aware that during the shutdown process, there are certain states that must be run for the SMO to properly shut itself (and this process) down. As such, one can add states to perform additional clean-ups, but should append the remaining state to be executed."
                # "SHUTTING DOWN"
                n109 = call <vilib>:"Add State(s) to Queue__jki_lib_state_machine.vi"("State(s) in (\"\")"=w317) -> ("States Out"=w316:string)  [unwired: 14 in]
              }
            }
            n110 = Bundle By Name(cluster=w304, "Core.Last Error.error"=w309) -> (w305:T8)
            n111 = call <vilib>:"Add State(s) to Queue__jki_lib_state_machine.vi"("State(s) in Front (\"\")"=w303, "State(s) in (\"\")"=w314) -> ("States Out"=w313:string)  [unwired: 13 in]
          }
          frame "Macro: Read UI Config" {
            # "Do not put any code in this frame.\n(It is a separator no-op. You can make a copy of this frame to create a new Macro frame)"
            n112 = call <vilib>:"Add State(s) to Queue__jki_lib_state_machine.vi"("State(s) in Front (\"\")"="Configuration: Initialize\nConfiguration: Read UI Config File\nUI: Update FP Controls" ("State(s) in Front (\"\")"), "State(s) in (\"\")"=w324) -> ("States Out"=w323:string)  [unwired: 13 in]
          }
          frame "Macro: Write UI Config" {
            # "Do not put any code in this frame.\n(It is a separator no-op. You can make a copy of this frame to create a new Macro frame)"
            n113 = call <vilib>:"Add State(s) to Queue__jki_lib_state_machine.vi"("State(s) in Front (\"\")"="Data: Set UI Cluster\nConfiguration: Write UI Config File" ("State(s) in Front (\"\")"), "State(s) in (\"\")"=w330) -> ("States Out"=w329:string)  [unwired: 13 in]
          }
          frame "Macro: Exit" {
            # "Exit Macro\n(This is called once, when the VI exits)"
            n114 = Unbundle By Name(w332) -> ("Core.Close Panel on Exit?"=w342:bool)
            n115 = Select(t="UI: Front Panel State >> Close", s=w342, f="" ("Empty String Constant")) -> (s? t:f=w339:string)
            n116 = call <vilib>:"Add State(s) to Queue__jki_lib_state_machine.vi"("State(s) in Front (\"\")"="Data: Cleanup\nEvents: Unregister\nProcess: Self Terminate", "State(s) in (\"\")"="Process: Sync", "State(s) at Back (\"\")"="Exit") -> ("States Out"=w334:string)  [unwired: 12 in]
            n117 = call <vilib>:"Add State(s) to Queue__jki_lib_state_machine.vi"("State(s) in Front (\"\")"="Action: Close\nMacro: Write UI Config", "State(s) in (\"\")"=w339, "State(s) at Back (\"\")"=w334) -> ("States Out"=w338:string)  [unwired: 12 in]
            n118 = call <vilib>:"Add State(s) to Queue__jki_lib_state_machine.vi"("State(s) in Front (\"\")"=w338, "State(s) in (\"\")"=w345) -> ("States Out"=w344:string)  [unwired: 13 in]
          }
          frame "---------- Process ----------" {
            # "Template Separator\n(You can make a copy of, or modify, this frame)"
            n119 = call <vilib>:"Add State(s) to Queue__jki_lib_state_machine.vi"("State(s) in (\"\")"=w350) -> ("States Out"=w349:string)  [unwired: 14 in]
          }
          frame "Process: Sync" {
            n120 = Unbundle By Name(w358) -> ("Instrument UI"=w354:refnum<class "Inst UI.SPC.lvclass">)
            n121 = call <vilib>:"WaitOnProcessSync.vi"("error in (no error)"=w353, "SMO"=w354) -> ("error out"=w352:errorcluster, "Don't run?"=w357:bool)  [unwired: 7 in, 1 out]
            n122 = Select(t="Data: Cleanup\nEvents: Unregister\nExit", s=w357, f="" ("Empty String Constant")) -> (s? t:f=w351:string)
            n123 = call <vilib>:"Add State(s) to Queue__jki_lib_state_machine.vi"("State(s) in Front (\"\")"=w351, "State(s) in (\"\")"=w361) -> ("States Out"=w360:string)  [unwired: 13 in]
          }
          frame "Process: Self Terminate" {
            n124 = Unbundle By Name(w363) -> ("Instrument UI"=w362:refnum<class "Inst UI.SPC.lvclass">)
            n125 = call <vilib>:"SelfTerminate.vi"("error in (no error)"=w365, "SMO in"=w362) -> ("error out"=w364:errorcluster)  [unwired: 8 in, 1 out]
            n126 = call <vilib>:"Add State(s) to Queue__jki_lib_state_machine.vi"("State(s) in (\"\")"=w368) -> ("States Out"=w367:string)  [unwired: 14 in]
          }
          frame "---------- Events ----------" {
            # "Template Separator\n(You can make a copy of, or modify, this frame)"
            n127 = call <vilib>:"Add State(s) to Queue__jki_lib_state_machine.vi"("State(s) in (\"\")"=w373) -> ("States Out"=w372:string)  [unwired: 14 in]
          }
          frame "Events: Register" {
            # "Expand to add\nmore events"
            # "Base Class Protected Events"
            n128 = Unbundle By Name(w387) -> ("Instrument UI"=w380:refnum<class "Inst UI.SPC.lvclass">, "Instrument"=w379:refnum<class "Inst.SPC.lvclass">)
            n129 = call <vilib>:"GetProtectedEvents.vi"("SMO"=w380) -> ("error out"=w383:errorcluster, "SMO Protected Events"=w385:T10)  [unwired: 8 in, 1 out]
            n130 = call <userlib>:"Instrument.GetPublicEvents.vi"("Instrument"=w379) -> ("error out"=w381:errorcluster, "Instrument Public Events"=w382:T11, "Instrument out"=w377:refnum<class "Inst.SPC.lvclass">)  [unwired: 8 in]
            n131 = call "Inst.SPC.GetPublicEvents.vi"("Inst.SPC in"=w377) -> ("error out"=w376:errorcluster, "Inst.SPC Public Events"=w378:T12)  [unwired: 8 in, 1 out]
            n132 = register-events(w385, w382, w378) -> (reference out=w386:refnum<event-registration>, error out=w375:errorcluster)  [unwired: 2 in]
            n133 = Merge Errors(w375, w376, w381, w383, w374) -> (w384:errorcluster)
            n134 = call <vilib>:"Add State(s) to Queue__jki_lib_state_machine.vi"("State(s) in (\"\")"=w389) -> ("States Out"=w388:string)  [unwired: 14 in]
          }
          frame "Events: Unregister" {
            n135 = Unregister For Events(event registration refnum=w392, error in=w391) -> (error out=w390:errorcluster)
            n136 = call <vilib>:"Add State(s) to Queue__jki_lib_state_machine.vi"("State(s) in (\"\")"=w395) -> ("States Out"=w394:string)  [unwired: 14 in]
          }
          frame "---------- Configuration ----------" {
            # "Do not put any code in this frame.\n(It is a separator no-op. You can make a copy of this frame to create a new UI frame)"
            n137 = call <vilib>:"Add State(s) to Queue__jki_lib_state_machine.vi"("State(s) in (\"\")"=w400) -> ("States Out"=w399:string)  [unwired: 14 in]
          }
          frame "Configuration: Initialize" {
            # "Do not put any code in this frame.\n(It is a separator no-op. You can make a copy of this frame to create a new UI frame)"
            n138 = Unbundle By Name(w408) -> ("Configuration"=w406:refnum<class "Configuration.lvclass">, "Instrument"=w407:refnum<class "Inst.SPC.lvclass">)
            n139 = call <vilib>:"GetName.vi"("error in (no error)"=w410, "SMO"=w407) -> ("error out"=w409:errorcluster, "Name"=w411:string)  [unwired: 6 in, 2 out]
            n140 = call <userlib>:"Default Path.vi"("error in (no error)"=w409, "Folder Name [Application Name]"=w411, "Configuration in"=w406) -> ("error out"=w402:errorcluster, "Configuration out"=w405:refnum<class "Configuration.lvclass">)  [unwired: 7 in]
            n141 = call <userlib>:"Write Section.vi"("error in (no error)"=w402, "Section"="UI", "Configuration in"=w405) -> ("error out"=w401:errorcluster, "Configuration out"=w404:refnum<class "Configuration.lvclass">)  [unwired: 7 in]
            n142 = Bundle By Name(cluster=w408, "Configuration"=w404) -> (w412:T8)
            n143 = call <vilib>:"Add State(s) to Queue__jki_lib_state_machine.vi"("State(s) in (\"\")"=w415) -> ("States Out"=w414:string)  [unwired: 14 in]
          }
          frame "Configuration: Write UI Config File" {
            # "Do not put any code in this frame.\n(It is a separator no-op. You can make a copy of this frame to create a new Data frame)"
            n144 = Unbundle By Name(w420) -> ("Configuration"=w417:refnum<class "Configuration.lvclass">, "UI Cluster"=w419:T6)
            n145 = call <userlib>:"Write Configuration.vi"("error in (no error)"=w416, "Variant"=w419, "Configuration in"=w417) -> ("error out"=w418:errorcluster)  [unwired: 7 in, 1 out]
            n146 = call <vilib>:"Add State(s) to Queue__jki_lib_state_machine.vi"("State(s) in (\"\")"=w423) -> ("States Out"=w422:string)  [unwired: 14 in]
          }
          frame "Configuration: Read UI Config File" {
            # "Do not put any code in this frame.\n(It is a separator no-op. You can make a copy of this frame to create a new UI frame)"
            n147 = Unbundle By Name(w426) -> ("UI Cluster"=w429:T6, "Configuration"=w432:refnum<class "Configuration.lvclass">)
            n148 = call <userlib>:"Read Configuration.vi"("INI Fomatted Cluster Type"=w429, "error in (no error)"=w428, "Configuration in"=w432) -> ("error out"=w431:errorcluster, "Configuration"=w430:variant)  [unwired: 6 in, 1 out]
            n149 = Variant To Data(error in=w431, type=w429, Variant=w430) -> (data=w425:T6, error out=w427:errorcluster)
            n150 = Bundle By Name(cluster=w426, "UI Cluster"=w425) -> (w424:T8)
            n151 = call <vilib>:"Add State(s) to Queue__jki_lib_state_machine.vi"("State(s) in (\"\")"=w435) -> ("States Out"=w434:string)  [unwired: 14 in]
          }
          frame "---------- Action ----------" {
            n152 = Unbundle By Name(w437) -> ("Instrument"=w438:refnum<class "Inst.SPC.lvclass">)
            n153 = Bundle By Name(cluster=w437, "Instrument"=w438) -> (w436:T8)
            n154 = call <vilib>:"Add State(s) to Queue__jki_lib_state_machine.vi"("State(s) in (\"\")"=w442) -> ("States Out"=w441:string)  [unwired: 14 in]
          }
          frame "Action: Notify UI Closed" {
            # "Notify that the UI has been closed"
            n155 = Unbundle By Name(w443) -> ("Instrument UI"=w446:refnum<class "Inst UI.SPC.lvclass">)
            n156 = call <vilib>:"Hide.vi"("error in (no error)"=w445, "SMO.UI"=w446) -> ("error out"=w444:errorcluster)  [unwired: 8 in, 1 out]
            n157 = call <vilib>:"Add State(s) to Queue__jki_lib_state_machine.vi"("State(s) in (\"\")"=w449) -> ("States Out"=w448:string)  [unwired: 14 in]
          }
          frame "Action: getAll" {
            n158 = Unbundle By Name(w453) -> ("getAll"=w451:T5, "Instrument"=w456:refnum<class "Inst.SPC.lvclass">)
            n159 = call "GET ALL.vim"("type"=w451, "error in (no error)"=w454, "Instrument in"=w456) -> ("error out"=w458:errorcluster, "getAll"=w450:T5, "Instrument out"=w452:refnum<class "Inst.SPC.lvclass">)  [unwired: 6 in]
            n160 = Bundle By Name(cluster=w453, "Instrument"=w452, "getAll"=w450) -> (w455:T8)
            n161 = call <vilib>:"Add State(s) to Queue__jki_lib_state_machine.vi"("State(s) in Front (\"\")"="" ("State(s) in Front (\"\")"), "State(s) in (\"\")"=w461) -> ("States Out"=w460:string)  [unwired: 13 in]
          }
          frame "Action: Open" {
            n162 = Unbundle By Name(w468) -> ("Instrument"=w466:refnum<class "Inst.SPC.lvclass">)
            n163 = call <userlib>:"Write Client Type.vi"("error in (no error)"=w463, "Client Type"=Client_Type--Enum."Local", "Instrument in"=w466) -> ("error out"=w464:errorcluster, "Instrument out"=w465:refnum<class "Inst.SPC.lvclass">)  [unwired: 7 in]
            n164 = call-dynamic "Open.vi"("error in (no error)"=w464, "Inst.SPC in"=w465) -> ("error out"=w471:errorcluster, "Inst.SPC out"=w467:refnum<class "Inst.SPC.lvclass">)  [unwired: 8 in]
            n165 = Bundle By Name(cluster=w468, "Instrument"=w467) -> (w469:T8)
            n166 = call <vilib>:"Add State(s) to Queue__jki_lib_state_machine.vi"("State(s) in Front (\"\")"="" ("State(s) in Front (\"\")"), "State(s) in (\"\")"=w474) -> ("States Out"=w473:string)  [unwired: 13 in]
          }
          frame "Action: Close" {
            n167 = Unbundle By Name(w476) -> ("Instrument"=w479:refnum<class "Inst.SPC.lvclass">)
            n168 = call-dynamic "Close.vi"("error in (no error)"=w477, "Inst.SPC in"=w479) -> ("error out"=w481:errorcluster, "Inst.SPC out"=w475:refnum<class "Inst.SPC.lvclass">)  [unwired: 8 in]
            n169 = Bundle By Name(cluster=w476, "Instrument"=w475) -> (w478:T8)
            n170 = call <vilib>:"Add State(s) to Queue__jki_lib_state_machine.vi"("State(s) in Front (\"\")"="" ("State(s) in Front (\"\")"), "State(s) in (\"\")"=w484) -> ("States Out"=w483:string)  [unwired: 13 in]
          }
          frame "Action: Send Message to Instrument" {
            # "Send a message (command, data, etc) to the Instrument:process.vi"
            n171 = Unbundle By Name(w489) -> ("Instrument"=w488:refnum<class "Inst.SPC.lvclass">)  [unwired: 1 out]
            n172 = call <userlib>:"Instrument.MessageToProcess.vi"("error in (no error)"=w486, "Instrument"=w488) -> ("error out"=w485:errorcluster, "Instrument out"=w487:refnum<class "Inst.SPC.lvclass">)  [unwired: 8 in]
            n173 = Bundle By Name(cluster=w489, "Instrument"=w487) -> (w490:T8)
            n174 = call <vilib>:"Add State(s) to Queue__jki_lib_state_machine.vi"("State(s) in Front (\"\")"="" ("State(s) in Front (\"\")"), "State(s) in (\"\")"=w494) -> ("States Out"=w493:string)  [unwired: 13 in]
          }
          frame "Action: Send Message to Child" {
            # "Send a message (command, data, etc) to the Instrument.Child:process.vi"
            n175 = Unbundle By Name(w499) -> ("Instrument"=w498:refnum<class "Inst.SPC.lvclass">)  [unwired: 1 out]
            n176 = call "Inst.SPC.MessageToProcess.vi"("error in (no error)"=w496, "Inst.SPC in"=w498) -> ("error out"=w495:errorcluster, "Inst.SPC out"=w497:refnum<class "Inst.SPC.lvclass">)  [unwired: 8 in]
            n177 = Bundle By Name(cluster=w499, "Instrument"=w497) -> (w500:T8)
            n178 = call <vilib>:"Add State(s) to Queue__jki_lib_state_machine.vi"("State(s) in Front (\"\")"="" ("State(s) in Front (\"\")"), "State(s) in (\"\")"=w504) -> ("States Out"=w503:string)  [unwired: 13 in]
          }
          frame "Action: GetConfig" {
            # "Send a message (command, data, etc) to the Instrument.Child:process.vi"
            n179 = Unbundle By Name(w511) -> ("Instrument"=w509:refnum<class "Inst.SPC.lvclass">)
            n180 = call <userlib>:"Instrument.MessageToProcess.vi"("error in (no error)"=w506, "Command"="GetConfig", "Instrument"=w509) -> ("error out"=w505:errorcluster, "Instrument out"=w507:refnum<class "Inst.SPC.lvclass">)  [unwired: 7 in]
            n181 = Bundle By Name(cluster=w511, "Instrument"=w507) -> (w510:T8)
            n182 = call <vilib>:"Add State(s) to Queue__jki_lib_state_machine.vi"("State(s) in Front (\"\")"="" ("State(s) in Front (\"\")"), "State(s) in (\"\")"=w515) -> ("States Out"=w514:string)  [unwired: 13 in]
          }
        }
      }
    }
    frame Error {
    }
  }
  n183 = call-parent "Process.vi"("error in"=w5, "Instrument UI in"=w4) -> ("error out"=w2:errorcluster, "Instrument UI out"=→"Inst UI.SPC out":refnum<class "Inst UI.SPC.lvclass">)  [unwired: 8 in]
  n184 = Merge Errors(w2, w1) -> (→"error out":errorcluster)
